vi "Get Recipe Status.vi"(8 "error in (no error)":errorcluster, 11 "Recipe Controller in":refnum<class "Recipe Controller.lvclass">) -> (0 "error out":errorcluster, 2 "Recipe State Data":refnum<data-value>, 3 "Recipe Controller out":refnum<class "Recipe Controller.lvclass">)   [LabVIEW 2022 SP3, in "Recipe Controller.lvclass"]
uses:
  Recipe Controller.lvclass
  Recipe Controller.lvclass/Recipe Controller.ctl
  Recipe State Data/Recipe State Data.lvclass
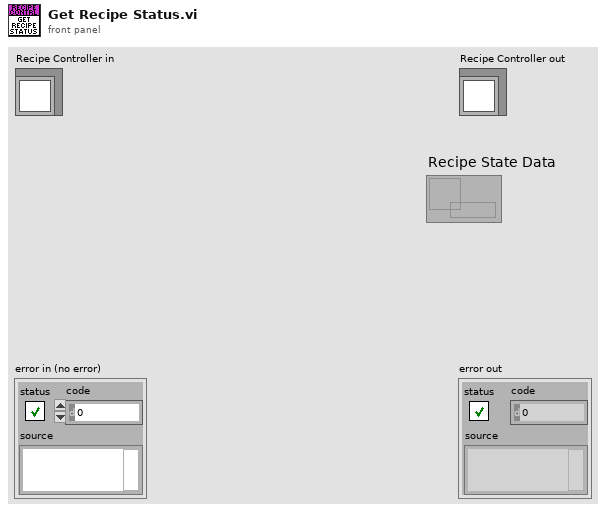
[diagram p1: front panel]
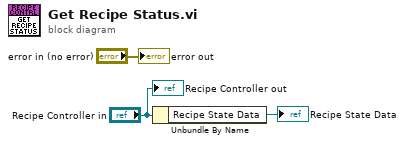
[diagram p0: block diagram]
diagram:
  n1 = Unbundle By Name("Recipe Controller in") -> ("Recipe State Data"=→"Recipe State Data":refnum<data-value>)
  "error out" <- "error in (no error)"
  "Recipe Controller out" <- "Recipe Controller in"
